vi "Read Constraints.vi"(8 "error in (no error)":errorcluster, 11 "Binary Operator in":refnum<class "Binary Operator.lvclass">) -> (0 "error out":errorcluster, 2 "Constraints":refnum<class "Constraint.lvclass">[](array[class]), 3 "Binary Operator out":refnum<class "Binary Operator.lvclass">)   [LabVIEW 2017, in "Transparent Assertions.lvlib" / "Binary Operator.lvclass"]
uses:
  Binary Operator.lvclass
  Constraint/Constraint.lvclass
  Binary Operator.lvclass/Binary Operator.ctl
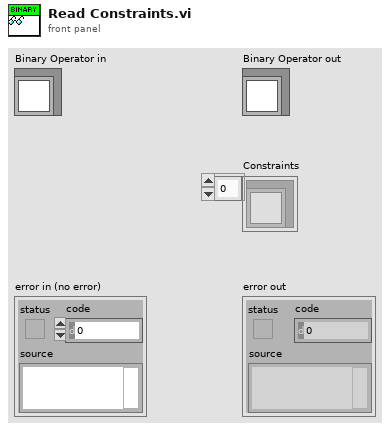
[diagram p1: front panel]
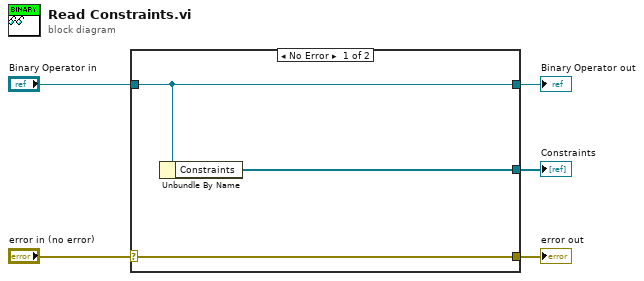
[diagram p0: block diagram]
diagram:
  n1 = case shown="No Error" "error in (no error)" {
    selector: "error in (no error)" -> [w8 w9]
    tunnel: [w8 w9] -> w4
    tunnel: [w7 w10] -> w2
    tunnel: "Binary Operator in" -> [w7 w10]
    tunnel: [w6 _] -> w1
    frame No Error {
      n2 = Unbundle By Name(w7) -> ("Constraints"=w6:refnum<class "Constraint.lvclass">[])
    }
    frame Error {
    }
  }
  "error out" <- w4
  "Binary Operator out" <- w2
  "Constraints" <- w1
